vi "Write Temp Stable.vi"(8 "error in (no error)":errorcluster, 10 "Temp Stable":bool, 11 "mTEC Data in":refnum<class "mTEC Data.lvclass">) -> (0 "error out":errorcluster, 3 "mTEC Data out":refnum<class "mTEC Data.lvclass">)   [LabVIEW 2014, in "Meerstetter Lib.lvlib" / "mTEC Data.lvclass"]
uses:
  mTEC Data.lvclass
  mTEC Data.lvclass/mTEC Data.ctl
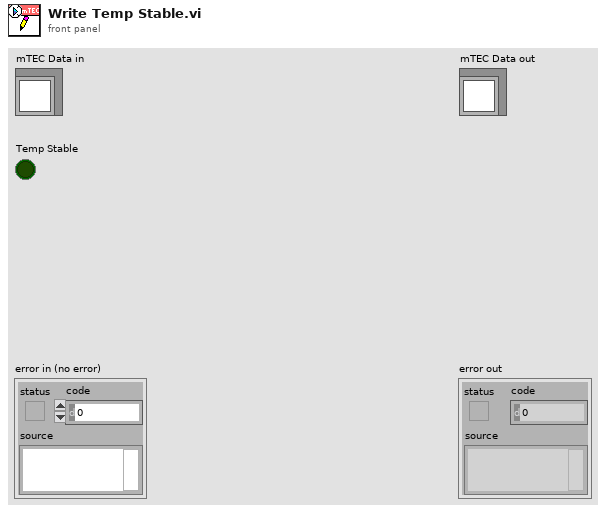
[diagram p1: front panel]
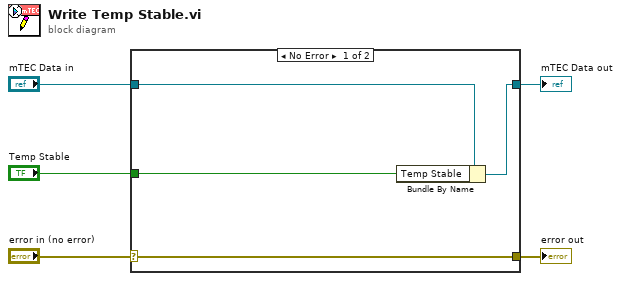
[diagram p0: block diagram]
diagram:
  n1 = case shown="No Error" "error in (no error)" {
    selector: "error in (no error)" -> [w9 w10]
    tunnel: [w9 w10] -> w4
    tunnel: [w7 w11] -> w2
    tunnel: "mTEC Data in" -> [w8 w11]
    tunnel: "Temp Stable" -> [w6 _]
    frame No Error {
      n2 = Bundle By Name(cluster=w8, "Temp Stable"=w6) -> (w7:refnum<class "mTEC Data.lvclass">)
    }
    frame Error {
    }
  }
  "error out" <- w4
  "mTEC Data out" <- w2
